vi "General Cosine Window (DBL).vi"(2 "Cosine Coefficients":dbl[](array[numeric]), 3 "X":dbl[](array[numeric])) -> (0 "error":i32, 1 "Windowed X":dbl[](array[numeric]))   [LabVIEW 2018, in "NI_AALPro.lvlib"]
doc: "Applies a general cosine window to the input signal <B>X</B>. Wire data to the <B>X</B> input to determine the polymorphic instance to use or manually select the instance."
uses:
  NI_AALPro.lvlib
  <resource>/lvanlys.dll
panel:
  # "General Cosine Window"
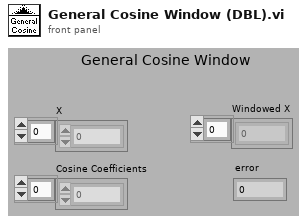
[diagram p1: front panel]
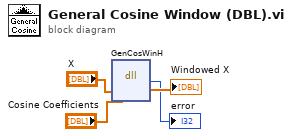
[diagram p0: block diagram]
diagram:
  n1 = dll-call lib="C:/Program Files (x86)/National Instruments/LabVIEW 2018/resource/lvanlys.*" fn="GenCosWinH"("X"="X", "Cosine Coefficients"="Cosine Coefficients") -> (→"error":i32, "X"=→"Windowed X":dbl[])  [unwired: 4 in, 2 out]
